vi "ThisIsATest.vi"() -> ()   [LabVIEW 2016]
panel:
  in  "true/false clock":bool
  in  "stop 2":bool
  out "diff":dbl
  out "Numeric":dbl
  out "Numeric 2":dbl
  in  "PUSH":bool
  in  "stop":bool
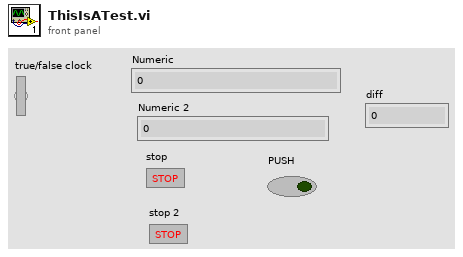
[diagram p1: front panel]
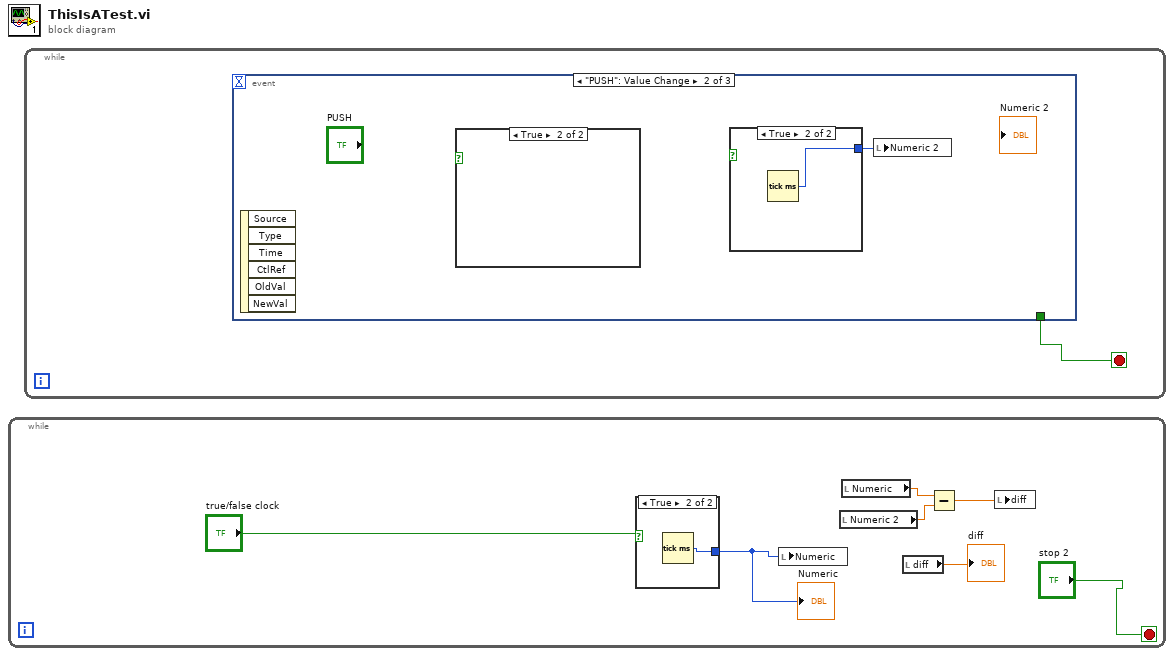
[diagram p0: block diagram]
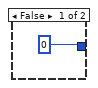
[diagram p2: hidden frame]
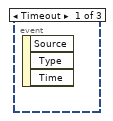
[diagram p3: hidden frame]
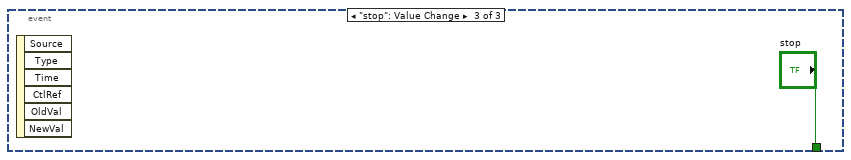
[diagram p6: hidden frame]
diagram:
  n1 = while {
    stop <- "stop 2" stop-if-true
    n2 = case shown="True" "true/false clock" {
      tunnel: [0 w9] -> w7
      frame False {
      }
      frame True {
        n3 = Tick Count (ms)() -> (millisecond timer value=w9:u32)
      }
    }
    "Numeric" <- w7
    n4 = local write "Numeric"(w7) -> ()
    n5 = local read "Numeric 2"() -> (w5:dbl)
    n6 = local read "Numeric"() -> (w6:dbl)
    n7 = local read "diff"() -> (→"diff":dbl)
    n8 = Subtract(x=w6, y=w5) -> (x-y=w4:dbl)
    n9 = local write "diff"(w4) -> ()
  }
  n10 = while {
    stop <- w10 stop-if-true
    n11 = event shown="[1] \"PUSH\": Value Change" {
      selector: _ -> [_ _ _]
      dyn-events: _ -> [_ _ _]
      timeout: _ -> [_ _ _]
      tunnel: [_ _ "stop"] -> w10
      event Timeout {
        n12 = event-data() -> ()  [unwired: 1 in, 3 out]
      }
      event "PUSH": Value Change {
        n13 = event-data() -> ()  [unwired: 1 in, 6 out]
        n14 = case shown="True" {
          selector: _ -> [_ _]
          frame False {
          }
          frame True {
          }
        }
        n15 = case shown="True" {
          selector: _ -> [_ _]
          tunnel: [_ w12] -> w11
          frame False {
          }
          frame True {
            n16 = Tick Count (ms)() -> (millisecond timer value=w12:u32)
          }
        }
        n17 = local write "Numeric 2"(w11) -> ()
      }
      event "stop": Value Change {
        n18 = event-data() -> ()  [unwired: 1 in, 6 out]
      }
    }
  }
